vi "Exchanger.vi"(7 "득점팀":string, 8 "증가":i8, 9 "종목 선택":string) -> (3 "출력 문자열":string)   [LabVIEW 2020]
uses:
  var.vi
panel:
  out "현재 종목":string
  # "종목, 증가점수, 득점팀 등을 입력받아 적절한 문장을 만들어내는 subVI"
  # "2017243031 최주홍"
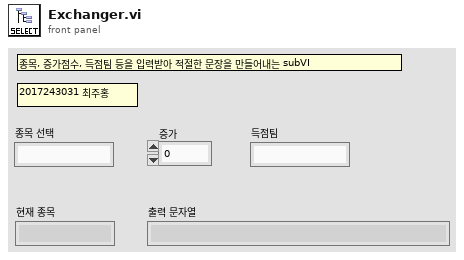
[diagram p1: front panel]
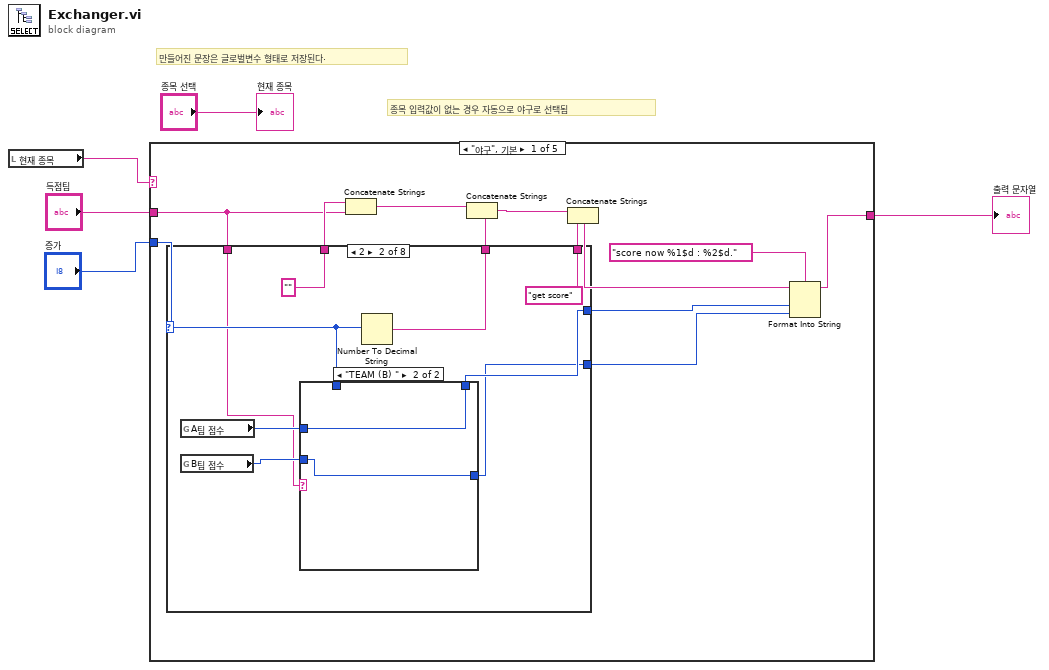
[diagram p0: block diagram]
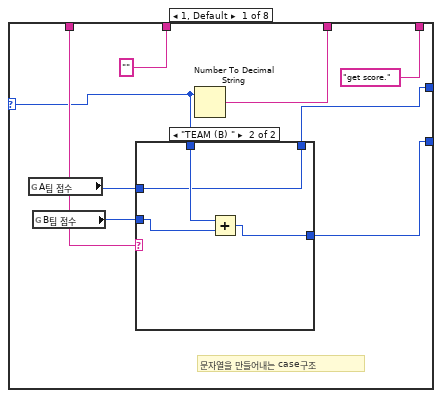
[diagram p2: hidden frame]
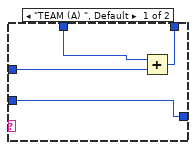
[diagram p3: hidden frame]
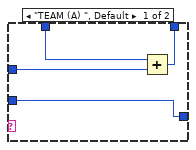
[diagram p4: hidden frame]
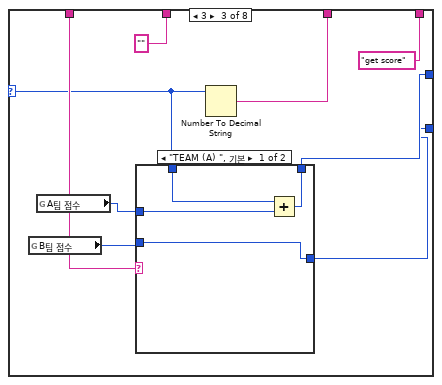
[diagram p5: hidden frame]
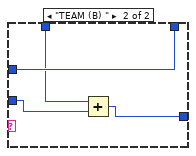
[diagram p6: hidden frame]
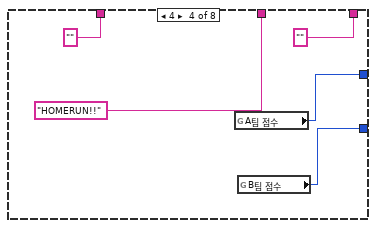
[diagram p7: hidden frame]
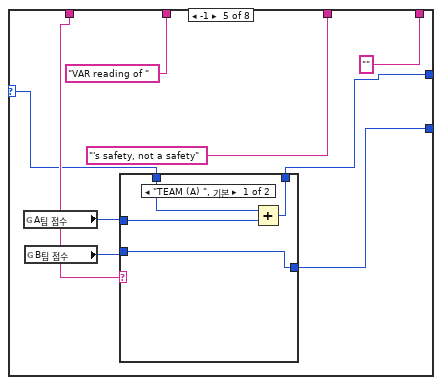
[diagram p8: hidden frame]
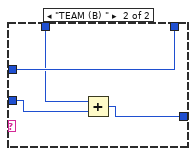
[diagram p9: hidden frame]
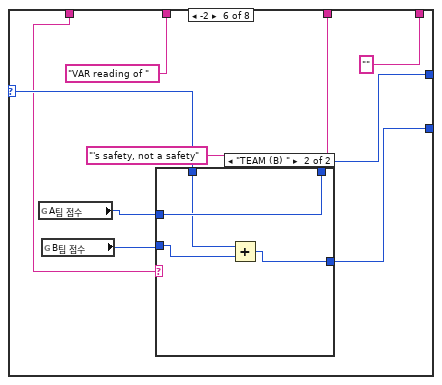
[diagram p10: hidden frame]
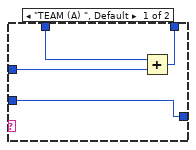
[diagram p11: hidden frame]
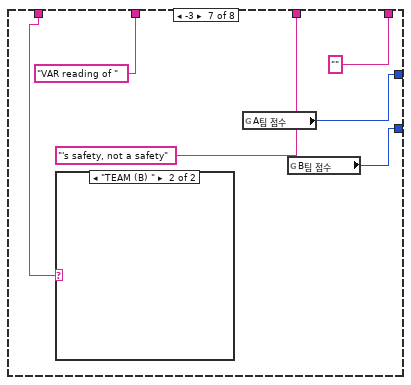
[diagram p12: hidden frame]
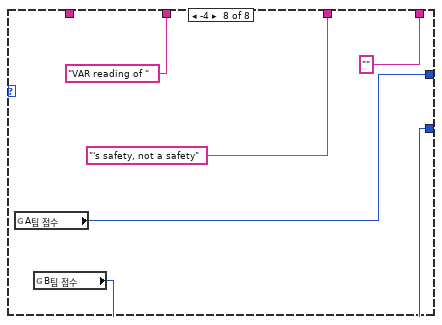
[diagram p14: hidden frame]
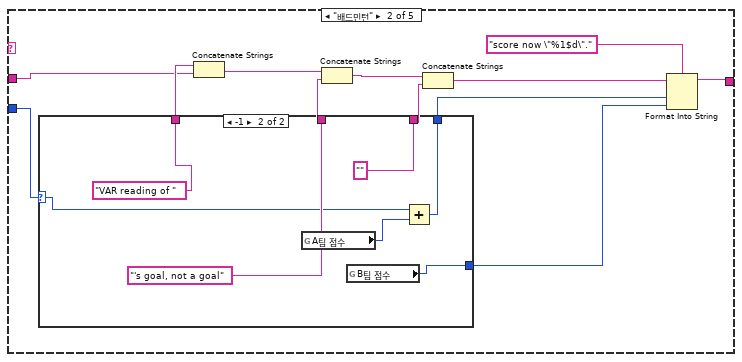
[diagram p15: hidden frame]
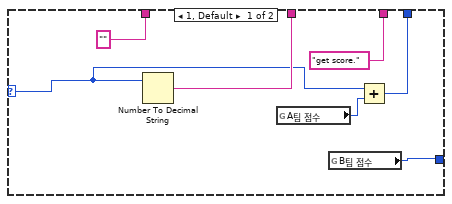
[diagram p16: hidden frame]
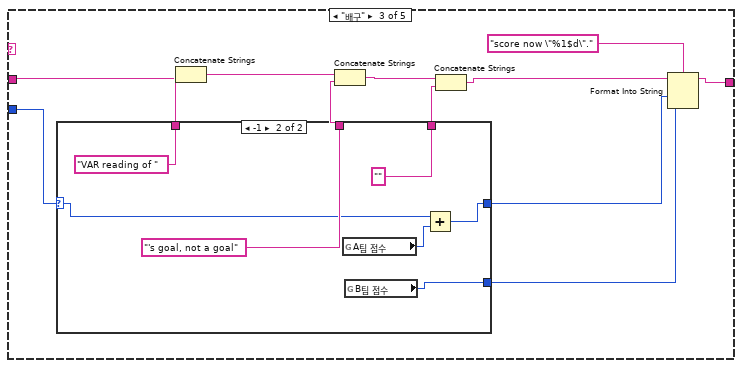
[diagram p17: hidden frame]
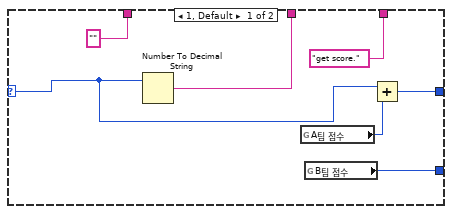
[diagram p18: hidden frame]
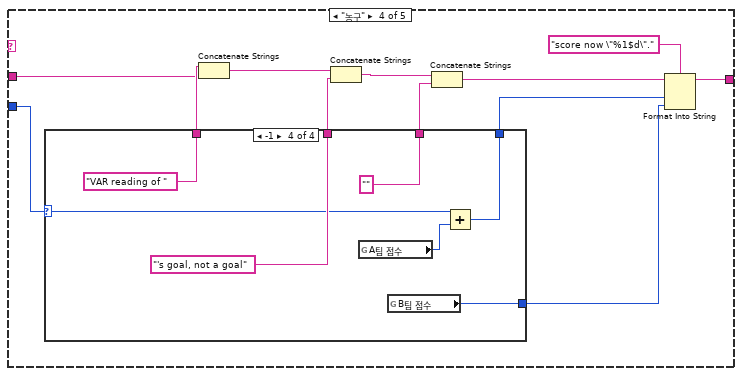
[diagram p19: hidden frame]
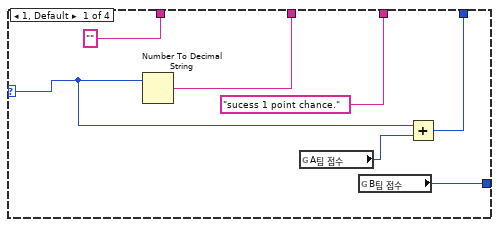
[diagram p20: hidden frame]
diagram:
  # "종목 입력값이 없는 경우 자동으로 야구로 선택됨"
  # "만들어진 문장은 글로벌변수 형태로 저장된다."
  n1 = local read "현재 종목"() -> (w3:string)
  n2 = case shown="\"야구\", 기본" w3 {
    tunnel: [w10 w121 w147 w173 w213] -> w5
    tunnel: "증가" -> [w9 w120 w146 w172 w211]
    tunnel: "득점팀" -> [w7 w119 w145 w171 w212]
    frame "야구", Default {
      n3 = case shown="2" w9 {
        selector: w9 -> [w21 w36 w54 _ w75 w94 _ _]
        tunnel: [w26 w43 w58 "HOMERUN!!" "'s safety, not a safety" "'s safety, not a safety" "'s safety, not a safety" "'s safety, not a safety"] -> w16
        tunnel: ["get score." "get score" "get score" "" "" "" "" ""] -> w15
        tunnel: ["" "" "" "" "VAR reading of " "VAR reading of " "VAR reading of " "VAR reading of "] -> w13
        tunnel: [w22 w38 w51 w67 w72 w90 w107 w113] -> w8
        tunnel: [w19 w37 w50 w68 w73 w89 w108 w112] -> w6
        tunnel: w7 -> [w23 w35 w55 _ w77 w91 w106 _]
        frame 1, Default {
          # "문자열을 만들어내는 case구조"
          n4 = global read "var.vi" "A팀 점수"() -> (w20:i8)
          n5 = global read "var.vi" "B팀 점수"() -> (w18:i8)
          n6 = case shown="\"TEAM (B) \"" w23 {
            tunnel: [w30 w31] -> w22
            tunnel: w21 -> [w29 w34]
            tunnel: w20 -> [w28 w31]
            tunnel: [w27 w32] -> w19
            tunnel: w18 -> [w27 w33]
            frame "TEAM (A) ", Default {
              n7 = Add(x=w29, y=w28) -> (x+y=w30:i8)
            }
            frame "TEAM (B) " {
              n8 = Add(x=w34, y=w33) -> (x+y=w32:i8)
            }
          }
          n9 = Number To Decimal String(number=w21) -> (decimal integer string=w26:string)  [unwired: 1 in]
        }
        frame 2 {
          n10 = global read "var.vi" "A팀 점수"() -> (w40:i8)
          n11 = global read "var.vi" "B팀 점수"() -> (w39:i8)
          n12 = case shown="\"TEAM (B) \"" w35 {
            tunnel: [w47 w49] -> w38
            tunnel: w40 -> [w46 w49]
            tunnel: [w45 w48] -> w37
            tunnel: w39 -> [w45 w48]
            tunnel: w36 -> [w44 _]
            frame "TEAM (A) ", Default {
              n13 = Add(x=w44, y=w46) -> (x+y=w47:i8)
            }
            frame "TEAM (B) " {
            }
          }
          n14 = Number To Decimal String(number=w36) -> (decimal integer string=w43:string)  [unwired: 1 in]
        }
        frame 3 {
          n15 = global read "var.vi" "B팀 점수"() -> (w52:i8)
          n16 = global read "var.vi" "A팀 점수"() -> (w53:i8)
          n17 = case shown="\"TEAM (A) \", 기본" w55 {
            tunnel: [w62 w64] -> w51
            tunnel: w53 -> [w61 w64]
            tunnel: [w60 w65] -> w50
            tunnel: w52 -> [w60 w66]
            tunnel: w54 -> [w59 w63]
            frame "TEAM (A) ", Default {
              n18 = Add(x=w59, y=w61) -> (x+y=w62:i8)
            }
            frame "TEAM (B) " {
              n19 = Add(x=w63, y=w66) -> (x+y=w65:i8)
            }
          }
          n20 = Number To Decimal String(number=w54) -> (decimal integer string=w58:string)  [unwired: 1 in]
        }
        frame 4 {
          n21 = global read "var.vi" "A팀 점수"() -> (w67:i8)
          n22 = global read "var.vi" "B팀 점수"() -> (w68:i8)
        }
        frame -1 {
          n23 = global read "var.vi" "A팀 점수"() -> (w76:i8)
          n24 = global read "var.vi" "B팀 점수"() -> (w74:i8)
          n25 = case shown="\"TEAM (A) \", 기본" w77 {
            tunnel: [w84 w86] -> w72
            tunnel: w76 -> [w83 w86]
            tunnel: [w82 w87] -> w73
            tunnel: w74 -> [w82 w88]
            tunnel: w75 -> [w81 w85]
            frame "TEAM (A) ", Default {
              n26 = Add(x=w81, y=w83) -> (x+y=w84:i8)
            }
            frame "TEAM (B) " {
              n27 = Add(x=w85, y=w88) -> (x+y=w87:i8)
            }
          }
        }
        frame -2 {
          n28 = global read "var.vi" "A팀 점수"() -> (w92:i8)
          n29 = global read "var.vi" "B팀 점수"() -> (w93:i8)
          n30 = case shown="\"TEAM (B) \"" w91 {
            tunnel: [w101 w103] -> w90
            tunnel: w92 -> [w100 w103]
            tunnel: [w99 w104] -> w89
            tunnel: w93 -> [w99 w105]
            tunnel: w94 -> [w98 w102]
            frame "TEAM (A) ", Default {
              n31 = Add(x=w98, y=w100) -> (x+y=w101:i8)
            }
            frame "TEAM (B) " {
              n32 = Add(x=w102, y=w105) -> (x+y=w104:i8)
            }
          }
        }
        frame -3 {
          n33 = case shown="\"TEAM (B) \"" w106 {
            frame "TEAM (A) ", Default {
            }
            frame "TEAM (B) " {
            }
          }
          n34 = global read "var.vi" "A팀 점수"() -> (w107:i8)
          n35 = global read "var.vi" "B팀 점수"() -> (w108:i8)
        }
        frame -4 {
          n36 = global read "var.vi" "A팀 점수"() -> (w113:i8)
          n37 = global read "var.vi" "B팀 점수"() -> (w112:i8)
        }
      }
      n38 = Concatenate Strings(w13, w7) -> (w14:string)
      n39 = Concatenate Strings(w14, w16) -> (w17:string)
      n40 = Concatenate Strings(w17, w15) -> (w11:string)
      n41 = Format Into String(format string="score now %1$d : %2$d.", initial string=w11, w8, w6) -> (resulting string=w10:string)  [unwired: 1 in, 1 out]
    }
    frame "배드민턴" {
      n42 = case shown="-1" w120 {
        selector: w120 -> [w130 w136]
        tunnel: [w135 "'s goal, not a goal"] -> w127
        tunnel: ["get score." ""] -> w126
        tunnel: ["" "VAR reading of "] -> w124
        tunnel: [w132 w139] -> w118
        tunnel: [w131 w138] -> w117
        frame 1, Default {
          n43 = Number To Decimal String(number=w130) -> (decimal integer string=w135:string)  [unwired: 1 in]
          n44 = global read "var.vi" "A팀 점수"() -> (w129:i8)
          n45 = global read "var.vi" "B팀 점수"() -> (w132:i8)
          n46 = Add(x=w130, y=w129) -> (x+y=w131:i8)
        }
        frame -1 {
          n47 = global read "var.vi" "A팀 점수"() -> (w137:i8)
          n48 = global read "var.vi" "B팀 점수"() -> (w139:i8)
          n49 = Add(x=w136, y=w137) -> (x+y=w138:i8)
        }
      }
      n50 = Concatenate Strings(w124, w119) -> (w125:string)
      n51 = Concatenate Strings(w125, w127) -> (w128:string)
      n52 = Concatenate Strings(w128, w126) -> (w122:string)
      n53 = Format Into String(format string="score now \"%1$d\".", initial string=w122, w117, w118) -> (resulting string=w121:string)  [unwired: 1 in, 1 out]
    }
    frame "배구" {
      n54 = case shown="-1" w146 {
        selector: w146 -> [w155 w162]
        tunnel: [w161 "'s goal, not a goal"] -> w153
        tunnel: ["get score." ""] -> w152
        tunnel: ["" "VAR reading of "] -> w150
        tunnel: [w156 w164] -> w144
        tunnel: [w158 w165] -> w143
        frame 1, Default {
          n55 = Number To Decimal String(number=w155) -> (decimal integer string=w161:string)  [unwired: 1 in]
          n56 = global read "var.vi" "A팀 점수"() -> (w157:i8)
          n57 = global read "var.vi" "B팀 점수"() -> (w158:i8)
          n58 = Add(x=w155, y=w157) -> (x+y=w156:i8)
        }
        frame -1 {
          n59 = global read "var.vi" "A팀 점수"() -> (w163:i8)
          n60 = global read "var.vi" "B팀 점수"() -> (w165:i8)
          n61 = Add(x=w162, y=w163) -> (x+y=w164:i8)
        }
      }
      n62 = Concatenate Strings(w150, w145) -> (w151:string)
      n63 = Concatenate Strings(w151, w153) -> (w154:string)
      n64 = Concatenate Strings(w154, w152) -> (w148:string)
      n65 = Format Into String(format string="score now \"%1$d\".", initial string=w148, w144, w143) -> (resulting string=w147:string)  [unwired: 1 in, 1 out]
    }
    frame "농구" {
      n66 = case shown="-1" w172 {
        selector: w172 -> [w181 w188 w195 w202]
        tunnel: [w187 w194 w201 "'s goal, not a goal"] -> w179
        tunnel: ["sucess 1 point chance." "sucess 2-point shot and get score." "sucess 3-point shot and get score." ""] -> w178
        tunnel: ["" "" "" "VAR reading of "] -> w176
        tunnel: [w183 w189 w197 w204] -> w170
        tunnel: [w184 w191 w198 w205] -> w169
        frame 1, Default {
          n67 = Number To Decimal String(number=w181) -> (decimal integer string=w187:string)  [unwired: 1 in]
          n68 = global read "var.vi" "A팀 점수"() -> (w182:i8)
          n69 = global read "var.vi" "B팀 점수"() -> (w184:i8)
          n70 = Add(x=w181, y=w182) -> (x+y=w183:i8)
        }
        frame 2 {
          n71 = Number To Decimal String(number=w188) -> (decimal integer string=w194:string)  [unwired: 1 in]
          n72 = global read "var.vi" "B팀 점수"() -> (w191:i8)
          n73 = global read "var.vi" "A팀 점수"() -> (w190:i8)
          n74 = Add(x=w188, y=w190) -> (x+y=w189:i8)
        }
        frame 3 {
          n75 = Number To Decimal String(number=w195) -> (decimal integer string=w201:string)  [unwired: 1 in]
          n76 = global read "var.vi" "A팀 점수"() -> (w196:i8)
          n77 = global read "var.vi" "B팀 점수"() -> (w198:i8)
          n78 = Add(x=w195, y=w196) -> (x+y=w197:i8)
        }
        frame -1 {
          n79 = global read "var.vi" "A팀 점수"() -> (w203:i8)
          n80 = global read "var.vi" "B팀 점수"() -> (w205:i8)
          n81 = Add(x=w202, y=w203) -> (x+y=w204:i8)
        }
      }
      n82 = Concatenate Strings(w176, w171) -> (w177:string)
      n83 = Concatenate Strings(w177, w179) -> (w180:string)
      n84 = Concatenate Strings(w180, w178) -> (w174:string)
      n85 = Format Into String(format string="score now \"%1$d\".", initial string=w174, w170, w169) -> (resulting string=w173:string)  [unwired: 1 in, 1 out]
    }
    frame "축구" {
      n86 = case shown="1, 기본" w211 {
        selector: w211 -> [w221 w228]
        tunnel: [w227 "'s goal, not a goal"] -> w218
        tunnel: ["get score." ""] -> w219
        tunnel: ["" "VAR reading of "] -> w216
        tunnel: [w223 w230] -> w210
        tunnel: [w224 w231] -> w209
        frame 1, Default {
          n87 = Number To Decimal String(number=w221) -> (decimal integer string=w227:string)  [unwired: 1 in]
          n88 = global read "var.vi" "A팀 점수"() -> (w222:i8)
          n89 = global read "var.vi" "B팀 점수"() -> (w224:i8)
          n90 = Add(x=w221, y=w222) -> (x+y=w223:i8)
        }
        frame -1 {
          n91 = global read "var.vi" "A팀 점수"() -> (w229:i8)
          n92 = global read "var.vi" "B팀 점수"() -> (w231:i8)
          n93 = Add(x=w228, y=w229) -> (x+y=w230:i8)
        }
      }
      n94 = Concatenate Strings(w216, w212) -> (w217:string)
      n95 = Concatenate Strings(w217, w218) -> (w220:string)
      n96 = Concatenate Strings(w220, w219) -> (w214:string)
      n97 = Format Into String(format string="score now \"%1$d\".", initial string=w214, w210, w209) -> (resulting string=w213:string)  [unwired: 1 in, 1 out]
    }
  }
  "출력 문자열" <- w5
  "현재 종목" <- "종목 선택"
